vi "Show With Fade In.vi"(8 "error in (no error)":errorcluster, 9 "Target Transparency (100)":u8=100, 10 "Fade time (800ms)":i32=800, 11 "Philips UI in":refnum<class "Flex UI.lvclass">) -> (0 "error out":errorcluster, 3 "Philips UI out":refnum<class "Flex UI.lvclass">)   [LabVIEW 2014, in "Flex UI.lvclass"]
uses:
  Flex UI.lvclass
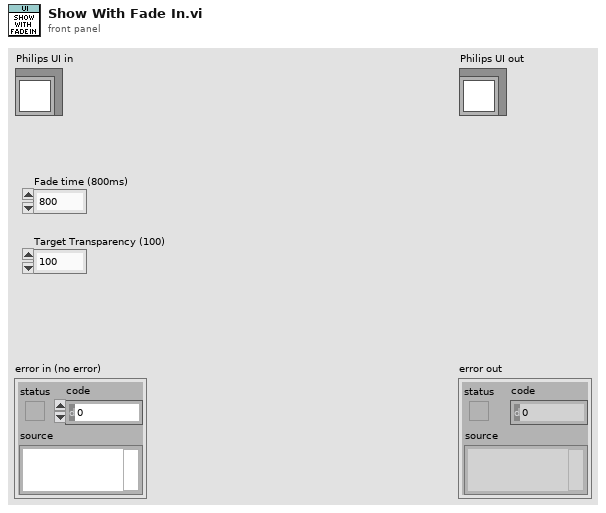
[diagram p1: front panel]
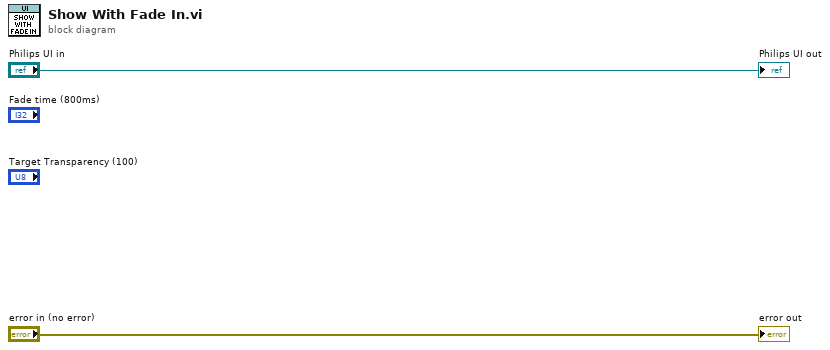
[diagram p0: block diagram]
diagram:
  "error out" <- "error in (no error)"
  "Philips UI out" <- "Philips UI in"
